vi "rewardJuicer.vi"(6 "seconds since 1Jan1904 2":timestamp, 7 "pulse dur":dbl, 8 "error in (no error)":errorcluster, 9 "IRI":dbl, 10 "Window Number (0...15)":i32, 11 "Juicer in":refnum<class "Juicer.lvclass">) -> (0 "error out":errorcluster, 1 "seconds since 1Jan1904":timestamp, 3 "Juicer out":refnum<class "Juicer.lvclass">)   [LabVIEW 2014, in "Juicer.lvclass"]
uses:
  Juicer.lvclass
  Juicer.lvclass/Juicer.ctl
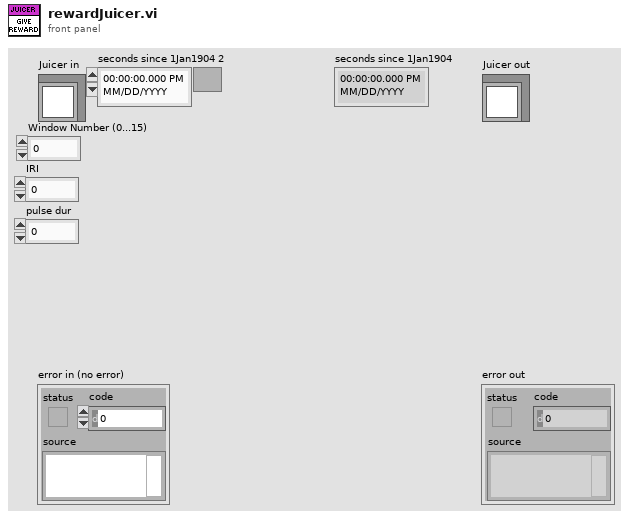
[diagram p1: front panel]
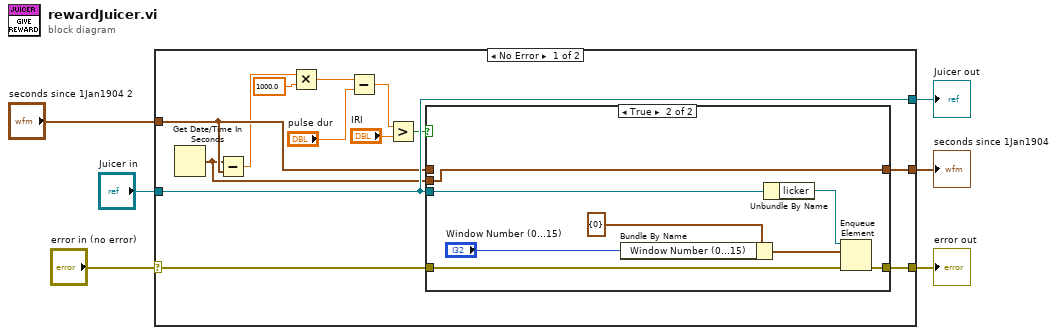
[diagram p0: block diagram]
diagram:
  n1 = case shown="No Error" "error in (no error)" {
    selector: "error in (no error)" -> [w19 w32]
    tunnel: [w18 w32] -> w5
    tunnel: [w16 w31] -> w3
    tunnel: "Juicer in" -> [w16 w31]
    tunnel: [w17 w30] -> w2
    tunnel: "seconds since 1Jan1904 2" -> [w15 w30]
    frame No Error {
      n2 = Get Date/Time In Seconds() -> (seconds since 1Jan1904=w14:timestamp)
      n3 = Subtract(x=w14, y=w15) -> (x-y=w11:dbl)
      n4 = Multiply(x=w11, y=1000.0) -> (x*y=w9:dbl)
      n5 = Subtract(x=w9, y="pulse dur") -> (x-y=w7:dbl)
      n6 = Greater?(x=w7, y="IRI") -> (0:w12:bool)
      n7 = case shown="True" w12 {
        tunnel: w16 -> [_ w29]
        tunnel: w19 -> [w20 w24]
        tunnel: [w20 w23] -> w18
        tunnel: [w21 w22] -> w17
        tunnel: w15 -> [w21 _]
        tunnel: w14 -> [_ w22]
        frame False {
        }
        frame True {
          n8 = Bundle By Name(cluster=cluster{"Window Number (0...15)":i32} {"Window Number (0...15)"=0} ("element"), "Window Number (0...15)"="Window Number (0...15)") -> (w26:cluster{"Window Number (0...15)":i32})
          n9 = Unbundle By Name(w29) -> ("licker"=w28:refnum<queue>)
          n10 = Enqueue Element(queue=w28, element=w26, error in (no error)=w24) -> (error out=w23:errorcluster)  [unwired: 1 in, 2 out]
        }
      }
    }
    frame Error {
    }
  }
  "error out" <- w5
  "Juicer out" <- w3
  "seconds since 1Jan1904" <- w2
